vi "OAT Config Color Map Indicator.vi"(0 "spectral map":dbl[][](array[numeric]) format="%.2f", 1 "color map ref":refnum<vi>, 5 "spectral map info":T1={"scales"={"x scale"={"offset"=0.0, "multiplier"=0.0}, "y scale"={"offset"=0.0, "multiplier"=0.0}}, "unit labels"={"x-axis unit label"="", "y-axis unit label"="", "z-axis unit label"=""}, "plot type"=enum."Frequency-Time", "dB on"=TRUE} {"scales"."y scale"."multiplier" format="%.2f"; "scales"."y scale"."offset" format="%.2f"; "scales"."x scale"."multiplier" format="%.2f"; "scales"."x scale"."offset" format="%.2f"}, 11 "error in (no error)":errorcluster) -> (4 "color map":T2, 15 "error out":errorcluster)   [LabVIEW 2017]
doc: "LabVIEW no longer supports this VI. Use the OAT Spectral Map VI instead. Configures the color map indicator and displays the vibration signal in the spectral map."
uses:
  <vilib>/addons/Sound and Vibration/Order Analysis/Backward Compatibility/SubVIs/OAT Spectral Map.ctl
  <vilib>/addons/Sound and Vibration/Order Analysis/Resample Order Tracking/SubVIs/Spectral Map Info.ctl
  <vilib>/addons/Sound and Vibration/Order Analysis/Resample Order Tracking/SoundVib_Resampling.lvlib
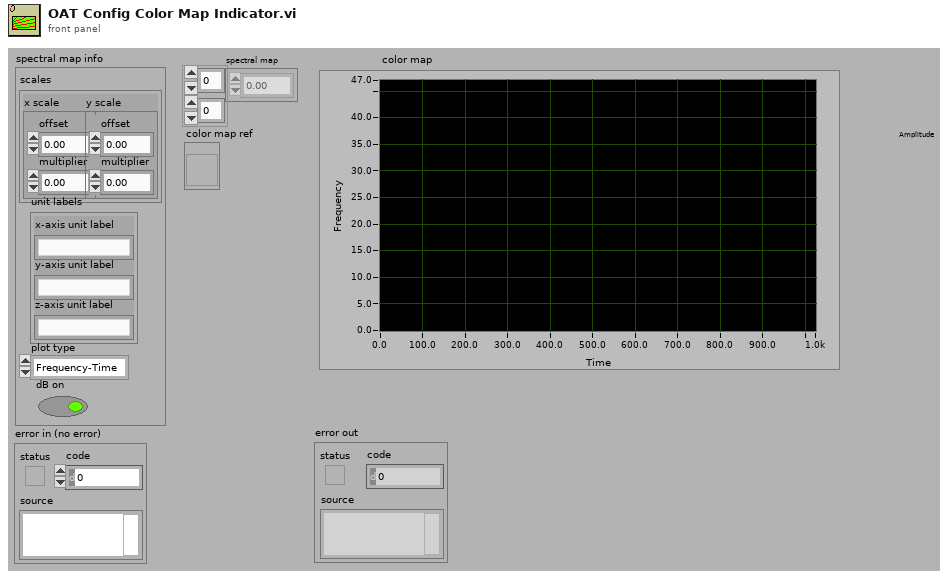
[diagram p1: front panel]
types:
  T1 = typedef "SoundVib_Resampling.lvlib/Spectral Map Info.ctl" = cluster{"scales":cluster{"x scale":cluster{"offset":dbl, "multiplier":dbl}, "y scale":cluster{"offset":dbl, "multiplier":dbl}}, "unit labels":cluster{"x-axis unit label":string, "y-axis unit label":string, "z-axis unit label":string}, "plot type":enum16{"Frequency-Time", "Time-Frequency", "Order-Time", "Time-Order", "Frequency-RPM", "RPM-Frequency", "Order-RPM", "RPM-Order"}, "dB on":bool}
  T2 = typedef "OAT Spectral Map.ctl" = dbl[][]
  T3 = cluster{"x scale":cluster{"offset":dbl, "multiplier":dbl}, "y scale":cluster{"offset":dbl, "multiplier":dbl}}
  T4 = cluster{"x-axis unit label":string, "y-axis unit label":string, "z-axis unit label":string}
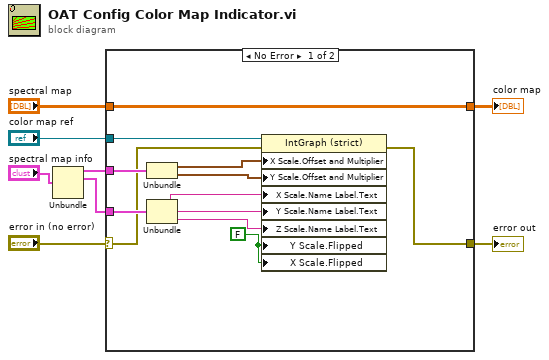
[diagram p0: block diagram]
diagram:
  n1 = Unbundle("spectral map info") -> ("scales"=w2:T3, "unit labels"=w1:T4)  [unwired: 2 out]
  n2 = case shown="No Error" "error in (no error)" {
    selector: "error in (no error)" -> [w13 w22]
    tunnel: [w12 w22] -> w7
    tunnel: "color map ref" -> [w20 _]
    tunnel: w2 -> [w19 _]
    tunnel: w1 -> [w17 _]
    tunnel: "spectral map" -> [w11 w21]
    tunnel: [w11 w21] -> w4
    frame No Error {
      w9 = FALSE ("Y Scale.Flipped")
      n3 = Unbundle(w19) -> ("x scale"=w18:cluster{"offset":dbl, "multiplier":dbl}, "y scale"=w10:cluster{"offset":dbl, "multiplier":dbl})
      n4 = Unbundle(w17) -> ("x-axis unit label"=w16:string, "y-axis unit label"=w15:string, "z-axis unit label"=w14:string)
      n5 = property class="IntGraph (strict)"(reference=w20, error in=w13, "X Scale.Offset and Multiplier"=w18, "Y Scale.Offset and Multiplier"=w10, "X Scale.Name Label.Text"=w16, "Y Scale.Name Label.Text"=w15, "Z Scale.Name Label.Text"=w14, "Y Scale.Flipped"=w9, "X Scale.Flipped"=w9) -> (error out=w12:errorcluster)  [unwired: 1 out]
    }
    frame Error {
    }
  }
  "color map" <- w4
  "error out" <- w7
